vi "DualTracker.vi"(6 "error in":errorcluster, 7 "XYZdata in":dbl[][][](array[numeric])) -> (1 "frame":i32, 4 "error in 2":errorcluster, 5 "XYZdata out":dbl[][][](array[numeric]))   [LabVIEW 2011]
panel:
  out "Debug output":sgl[][](graph)
  out "XY tracker difference":cluster{"[0]":dbl, "[1]":dbl}(graph)
  out "LV tracker rad prof":dbl[](graph)
  out "JTracker radial profile":sgl[](graph)
  out "1D xcor XY":cluster{"[0]":dbl, "[1]":dbl}(graph)
  out "Bead":i32
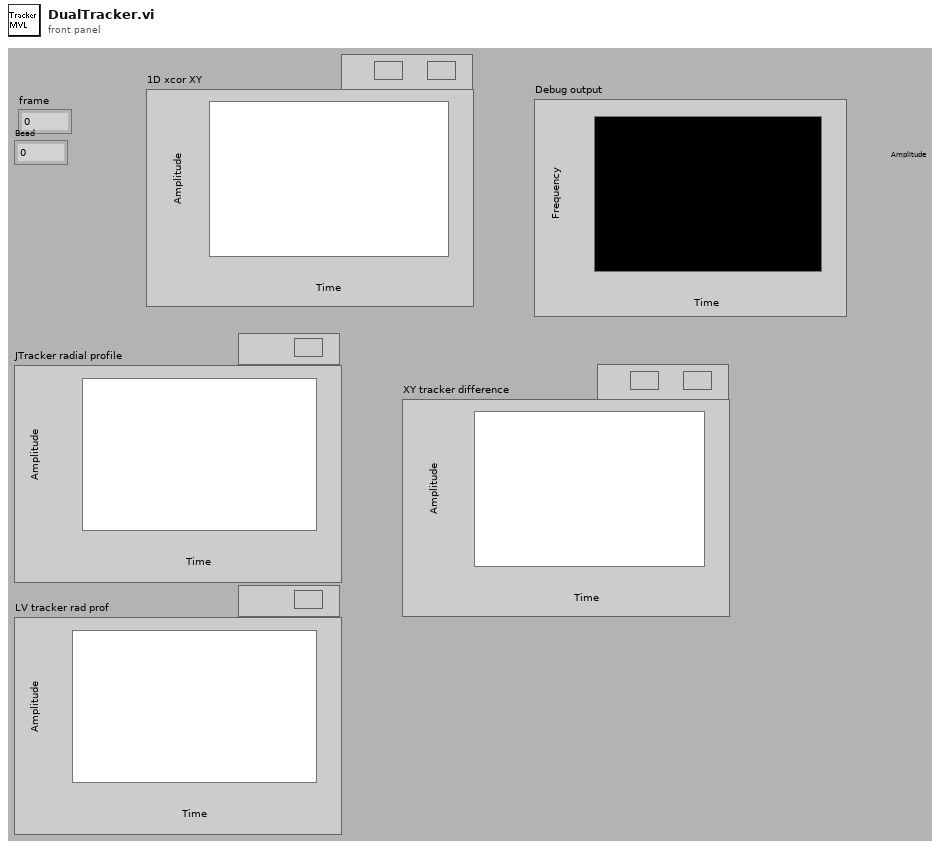
[diagram p1: front panel]
types:
  T1 = typedef "Image Type" = u32
  T2 = cluster{"Image Pixels (U8)":u8[][], "xy out":dbl[], "relative frame #":i32, "bead #":i32, "state":i32, "frame number":i32, "frame time":i32}
  T3 = cluster{"ROI1":i32, "Rmax (pix)":i32, "RminZ (pix)":i32, "LUTs":dbl[][][], "use trace":bool, "angular pixel\n coverage factor":dbl, "radial pixel\n coverage factor":dbl}
  T4 = typedef "IMAQ Image.ctl" = refnum<image>
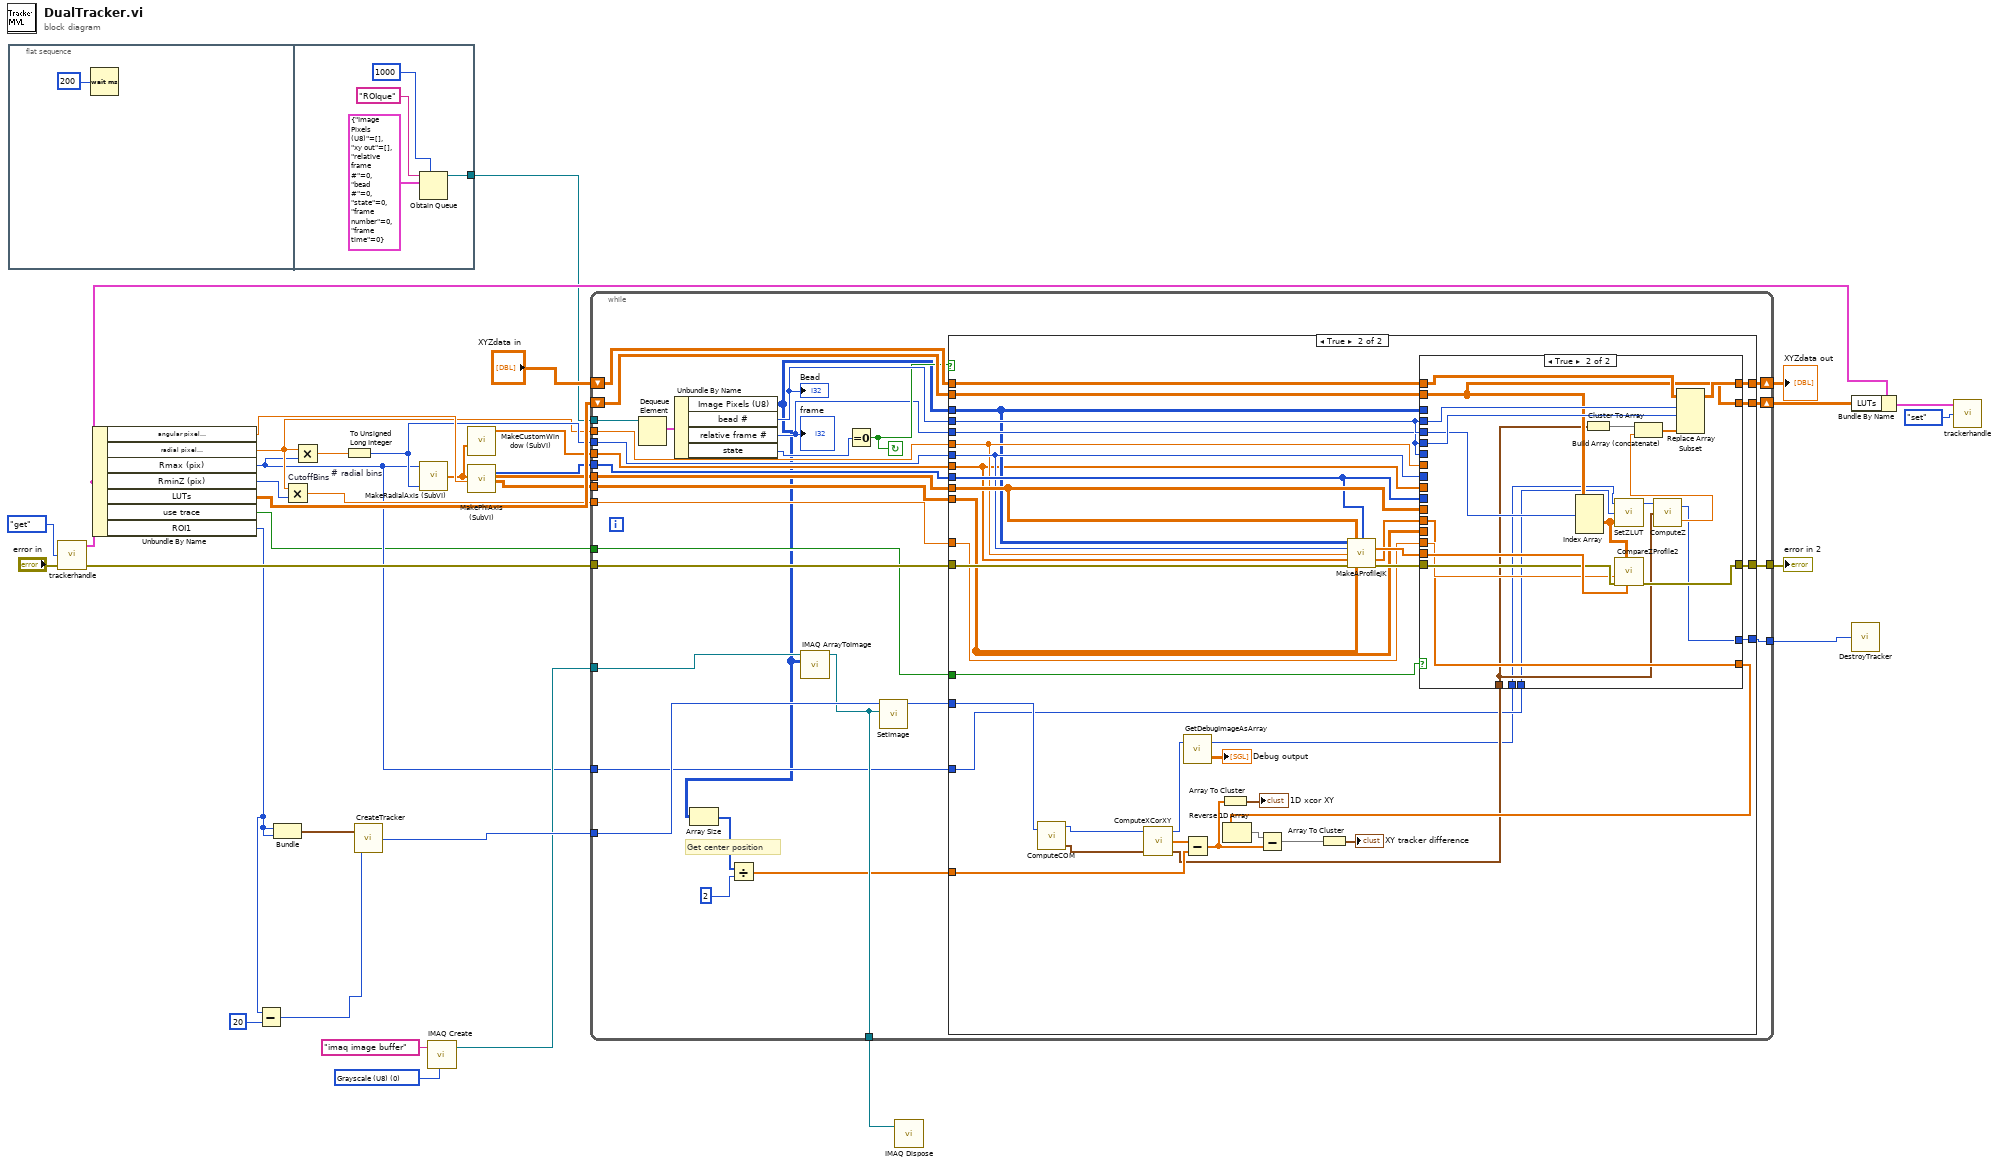
[diagram p0: block diagram]
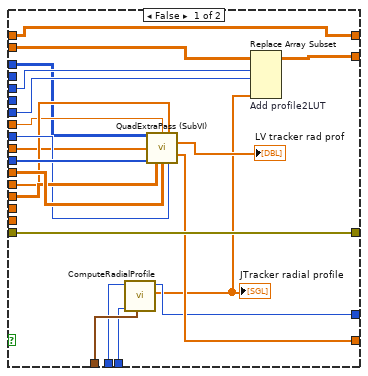
[diagram p3: hidden frame]
diagram:
  w9 = T1 0 items=["Grayscale (U8)", "Grayscale (I16)", "Grayscale (SGL)", "Complex (CSG)", "RGB (U32)", "HSL (U32)", "RGB (U64)", "Grayscale (U16)"] ("Image Type")
  n1 = flat-sequence {
    tunnel: [w38] -> w24
    frame #0 {
      n2 = Wait (ms)(milliseconds to wait=u32 200) -> ()  [unwired: 1 out]
    }
    frame #1 {
      n3 = Obtain Queue(max queue size (-1, unlimited)=1000, name (unnamed)="ROIque", element data type=T2 {"Image Pixels (U8)"=[], "xy out"=[], "relative frame #"=0, "bead #"=0, "state"=0, "frame number"=0, "frame time"=0} ("output cluster")) -> (queue out=w38:refnum<queue>)  [unwired: 2 in, 2 out]
    }
  }
  n4 = call "trackerhandle.vi"("error in"="error in", "action"=enum16{"get", "set"}."get") -> ("error out"=w26:errorcluster, "output Cluster"=w30:T3)  [unwired: 1 in, 1 out]
  n5 = Unbundle By Name(w30) -> ("angular pixel\n coverage factor"=w23:dbl, "radial pixel\n coverage factor"=w16:dbl, "Rmax (pix)"=w5:i32, "RminZ (pix)"=w15:i32, "LUTs"=w32:dbl[][][], "use trace"=w1:bool, "ROI1"=w2:i32)
  n6 = Subtract(x=w2, y=20) -> (x-y=w3:i32)
  n7 = Bundle("ROI1"=w2, "ROI1"=w2) -> (w12:cluster{"ROI1":i32, "ROI1":i32})  [unwired: 1 in]
  n8 = Multiply "CutoffBins"(x=w16, y=w15) -> (x*y=w14:dbl)
  n9 = Multiply(x=w16, y=w5) -> (x*y=w22:dbl)
  n10 = To Unsigned Long Integer "# radial bins"(number=w22) -> (unsigned 32bit integer=w20:u32)
  n11 = call "CreateTracker.vi"("XCorWindow"=w3, "Image size"=w12) -> ("return type"=w11:u64)
  n12 = call "MakeRadialAxis (SubVI).vi"("# radial bins"=w20, "Rmax-Rmin"=w5) -> ("radialaxis"=w21:dbl[])  [unwired: 1 in]
  n13 = call "IMAQ Create"("Image Name"="imaq image buffer", "Image Type"=w9) -> ("New Image"=w8:T4)  [unwired: 3 in, 1 out]
  n14 = call "MakeCustomWindow (SubVI).vi"("radialaxis"=w21) -> ("Halfstetson"=w13:dbl[])  [unwired: 8 in, 2 out]
  n15 = call "MakePhiAxis (SubVI).vi"("radialBinAxis"=w21, "angular pixel \ncoverage factor"=w23) -> ("lengths"=w19:i32[], "Rsin(phi)[Q]"=w18:dbl[][][], "Rcos(phi)[Q]"=w17:dbl[][][])  [unwired: 2 in, 13 out]
  n16 = while {
    shift-right: [w69] -> w33
    shift-left: "XYZdata in" -> [w68]
    shift-right: [w67] -> w28
    shift-left: w32 -> [w66]
    tunnel: w26 -> [w60]
    tunnel: [w59] -> w25
    tunnel: w24 -> [w62]
    tunnel: w16 -> [w61]
    tunnel: w20 -> [w57]
    tunnel: w19 -> [w56]
    tunnel: w18 -> [w55]
    tunnel: w17 -> [w54]
    tunnel: w13 -> [w53]
    tunnel: w14 -> [w52]
    tunnel: w11 -> [w51]
    tunnel: w8 -> [w50]
    tunnel: [w48] -> w7
    tunnel: [w47] -> w6
    tunnel: w1 -> [w46]
    tunnel: w5 -> [w45]
    stop <- w63 continue-if-true
    # "Get center position"
    n17 = Dequeue Element(queue=w62) -> (element=w70:T2)  [unwired: 1 in, 4 out]
    n18 = Unbundle By Name(w70) -> ("Image Pixels (U8)"=w43:u8[][], "bead #"=w64:i32, "relative frame #"=w58:i32, "state"=w65:i32)
    "frame" <- w58
    "Bead" <- w64
    n19 = Array Size(array=w43) -> (size(s)=w42:i32[])
    n20 = Divide(x=w42, y=2) -> (x/y=w41:dbl[])
    n21 = call "IMAQ ArrayToImage"("Image Pixels (U8)"=w43, "Image"=w50) -> ("Image Out"=w48:T4)  [unwired: 8 in, 1 out]
    n22 = Equal To 0?(x=w65) -> (x = 0?=w63:bool)
    n23 = call "SetImage.vi"("Image"=w48, "tracker"=w51) -> ("tracker"=w49:u64)  [unwired: 5 in]
    n24 = case shown="True" w63 {
      tunnel: [w74 w111] -> w69
      tunnel: w68 -> [w74 w110]
      tunnel: w64 -> [_ w109]
      tunnel: w58 -> [_ w108]
      tunnel: [w73 w107] -> w67
      tunnel: w66 -> [w73 w106]
      tunnel: w43 -> [_ w96]
      tunnel: w61 -> [_ w97]
      tunnel: w60 -> [w72 w104]
      tunnel: [w72 w102] -> w59
      tunnel: w57 -> [_ w98]
      tunnel: w56 -> [_ w99]
      tunnel: w55 -> [_ w100]
      tunnel: w54 -> [_ w101]
      tunnel: w53 -> [_ w94]
      tunnel: w52 -> [_ w95]
      tunnel: w49 -> [w71 w80]
      tunnel: [w71 w79] -> w47
      tunnel: w46 -> [_ w93]
      tunnel: w45 -> [_ w78]
      tunnel: w41 -> [_ w91]
      frame False {
      }
      frame True {
        n25 = call "ComputeCOM.vi"("tracker"=w80) -> ("tracker"=w89:u64, "position"=w88:cluster{"X":sgl, "Y":sgl})  [unwired: 1 in, 1 out]
        n26 = call "ComputeXCorXY.vi"("position"=w88, "tracker"=w89) -> ("position"=w81:cluster{"X":sgl, "Y":sgl}, "position array"=w87:sgl[], "tracker"=w77:u64)  [unwired: 1 in]
        n27 = call "GetDebugImageAsArray.vi"("tracker"=w77) -> ("image"=→"Debug output":sgl[][], "tracker"=w76:u64)  [unwired: 1 in]
        n28 = Subtract(x=w87, y=w91) -> (x-y=w84:dbl[])
        n29 = Array To Cluster(array=w84) -> (cluster=→"1D xcor XY":cluster{"[0]":dbl, "[1]":dbl})
        n30 = call "MakeAProfileJK.vi"("image in"=w96, "Rsin(phi)[Q]"=w100, "angularbinlengths"=w99, "# Radial bins"=w98, "radial bins/pixel"=w97, "window"=w94, "error in (no error) 2"=w104, "Rcos(phi)[Q]"=w101) -> ("radial profile"=w105:dbl[], "xy-out 1"=w92:dbl[], "error in (no error) 3"=w103:errorcluster)  [unwired: 3 in, 2 out]
        n31 = case shown="True" w93 {
          tunnel: w105 -> [_ w152]
          tunnel: w92 -> [w122 w141]
          tunnel: w110 -> [w132 w151]
          tunnel: w109 -> [_ w150]
          tunnel: w108 -> [_ w149]
          tunnel: [w132 w147] -> w111
          tunnel: w106 -> [w131 w145]
          tunnel: w109 -> [w130 w146]
          tunnel: w108 -> [w129 _]
          tunnel: [w128 w145] -> w107
          tunnel: w103 -> [w127 w144]
          tunnel: [w127 w143] -> w102
          tunnel: w101 -> [w125 _]
          tunnel: w100 -> [w126 _]
          tunnel: w99 -> [w124 _]
          tunnel: w98 -> [w123 _]
          tunnel: w97 -> [w121 _]
          tunnel: w96 -> [w120 _]
          tunnel: w95 -> [_ w142]
          tunnel: w94 -> [w119 _]
          tunnel: [w117 w141] -> w90
          tunnel: w81 -> [w116 w137]
          tunnel: w76 -> [w115 w136]
          tunnel: [w114 w139] -> w79
          tunnel: w78 -> [w113 w134]
          frame False {
            n32 = call "ComputeRadialProfile.vi"("center"=w116, "radius"=w113, "tracker"=w115) -> ("output"=w112:sgl[], "tracker"=w114:u64)  [unwired: 7 in]
            "JTracker radial profile" <- w112
            n33 = call "QuadExtraPass (SubVI).vi"("Image"=w120, "radial bins/pixel"=w121, "First position"=w122, "window"=w119, "angularbinlengths"=w124, "Rcos(phi)[Q]"=w125, "Rsin(phi)[Q]"=w126, "# Radial bins"=w123) -> ("radial profile"=→"LV tracker rad prof":dbl[], "New Position (pixels)"=w117:dbl[])  [unwired: 4 in, 2 out]
            n34 = Replace Array Subset "Add profile2LUT"(array=w131, new element=w112, index (dim 0)=w130, index (dim 1)=w129) -> (w128:dbl[][][])  [unwired: 1 in]
          }
          frame True {
            n35 = Index Array(array=w145, index (dim 0)=w146) -> (element=w133:dbl[][])  [unwired: 2 in]
            n36 = Cluster To Array(cluster=w137) -> (array=w138:sgl[])
            n37 = call "SetZLUT.vi"("zlut"=w133, "profile_radius"=w134, "tracker"=w136) -> ("tracker"=w135:u64)  [unwired: 2 in]
            n38 = call "CompareZProfile2.vi"("Z profile"=w152, "Z LUT"=w133, "error in 2"=w144, "Cutoff R(bins)"=w142) -> ("error out3"=w143:errorcluster)  [unwired: 6 out]
            n39 = call "ComputeZ.vi"("position"=w137, "tracker"=w135) -> ("Z"=w140:sgl, "tracker"=w139:u64)  [unwired: 1 in]
            n40 = Build Array (concatenate)(w138, w140) -> (w148:sgl[])
            n41 = Replace Array Subset(array=w151, new element=w148, index (dim 0)=w150, index (dim 1)=w149) -> (w147:dbl[][][])  [unwired: 1 in]
          }
        }
        n42 = Reverse 1D Array(array=w90) -> (reversed array=w85:dbl[])
        n43 = Subtract(x=w85, y=w84) -> (x-y=w83:dbl[])
        n44 = Array To Cluster(array=w83) -> (cluster=→"XY tracker difference":cluster{"[0]":dbl, "[1]":dbl})
      }
    }
  }
  "XYZdata out" <- w33
  "error in 2" <- w25
  n45 = call "IMAQ Dispose"("Image"=w7) -> ()  [unwired: 5 in, 1 out]
  n46 = Bundle By Name(cluster=w30, "LUTs"=w28) -> (w29:T3)
  n47 = call "DestroyTracker.vi"("tracker"=w6) -> ()
  n48 = call "trackerhandle.vi"("action"=enum16{"get", "set"}."set", "input Cluster"=w29) -> ()  [unwired: 1 in, 3 out]
